vi "Power_ctrl_to_ioEXPSET.vi"(8 "error in (no error)":errorcluster, 10 "IO exp. setting in":u16, 11 "Sensor power control":T1) -> (0 "error out":errorcluster, 2 "Sensor power out":T1, 3 "IO expaneder setting out":u16 format="%x")   [LabVIEW 2013]
doc: "Conversion VI between sent data to control power to sensors and sensor intefaces. \nSet which sensors should be powered in cluster, get coverted bool array using this vi, send to unit.\nGet status from unit, convert it using this VI to cluster where you see which sensors are powered.\n\nBool array is useless, updated to uint16 input/output"
uses:
  Sensor_power_ctrl.ctl
panel:
  out "Boolean array":bool[](array[boolean])
  out "size(s) 2":i32
  out "size(s)":i32
  in  "lookup port":u16[](array[numeric])=[3, 2, 6, 7, 14, 15, 4, 5, 1, 0] format="%0d"
  out "Bool Array out":bool[](array[boolean])
  # "power control to bool array"
  # "index is power control in order\nvalue is specific IOexp output\nordered 0 is 0.0, 7 is 0.7, 8 is 1.0 15 is 1.7"
  # "8"
  # "old values"
  # "bool array to power control"
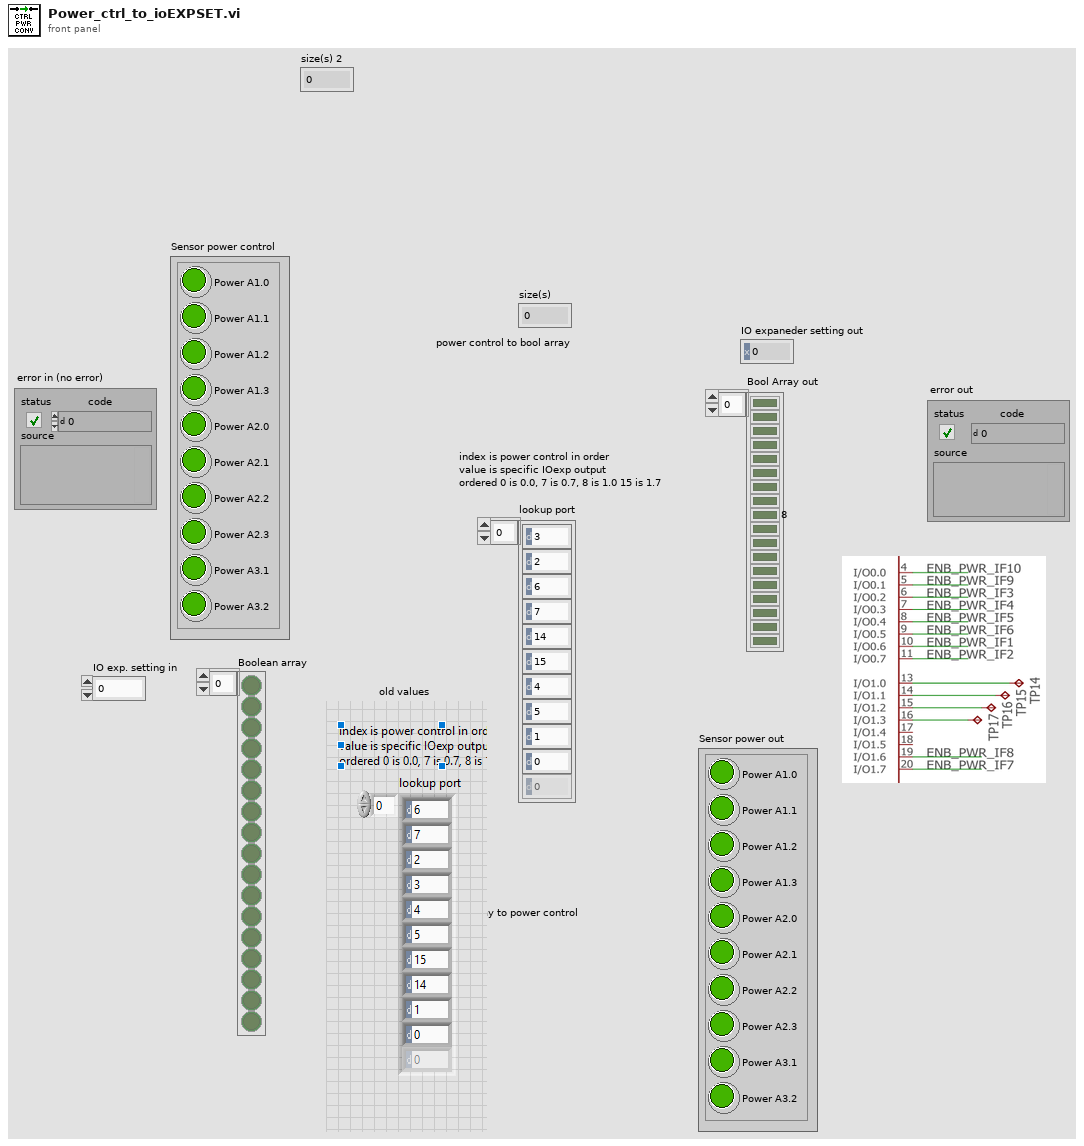
[diagram p1: front panel]
types:
  T1 = typedef "Sensor_power_ctrl.ctl" = cluster{"Power A1.0":bool, "Power A1.1":bool, "Power A1.2":bool, "Power A1.3":bool, "Power A2.0":bool, "Power A2.1":bool, "Power A2.2":bool, "Power A2.3":bool, "Power A3.1":bool, "Power A3.2":bool}
  T2 = cluster{"[0]":bool, "[1]":bool, "[2]":bool, "[3]":bool, "[4]":bool, "[5]":bool, "[6]":bool, "[7]":bool, "[8]":bool, "[9]":bool}
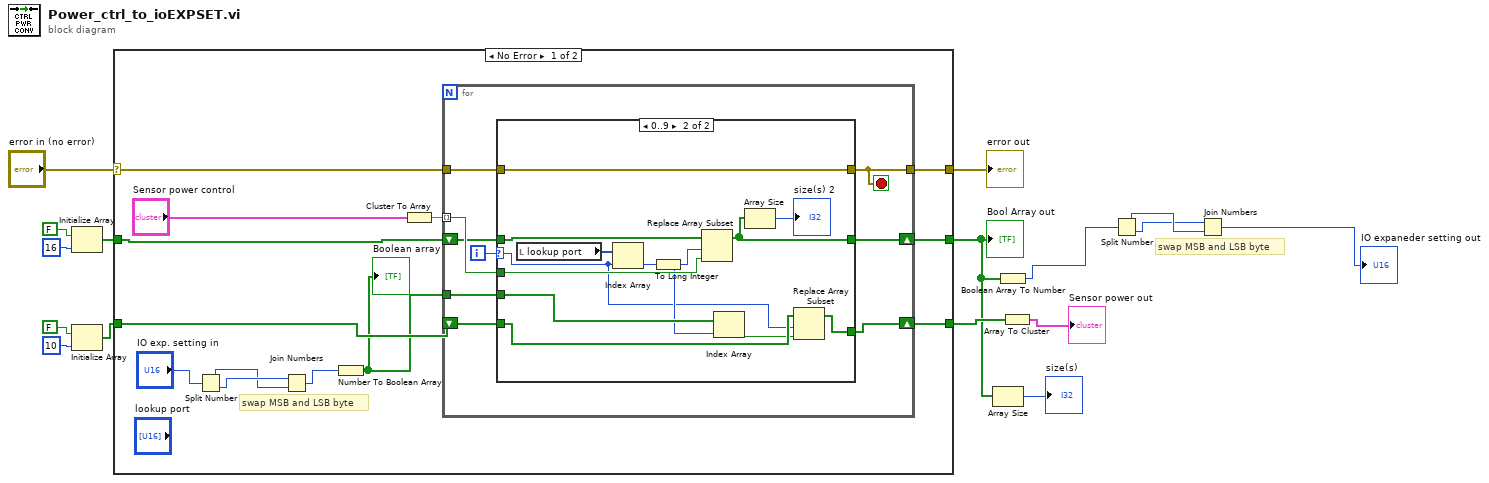
[diagram p0: block diagram]
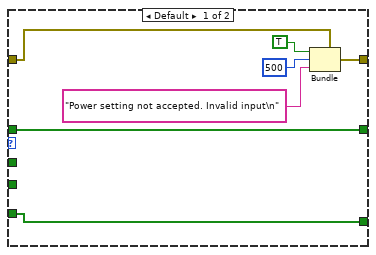
[diagram p2: hidden frame]
diagram:
  # "swap MSB and LSB byte"
  n1 = Initialize Array(FALSE, 16 ("dimension size")) -> (w12:bool[])
  n2 = Initialize Array(FALSE, 10 ("dimension size")) -> (w8:bool[])
  n3 = case shown="No Error" "error in (no error)" {
    selector: "error in (no error)" -> [w29 w60]
    tunnel: [w28 w60] -> w15
    tunnel: w12 -> [w27 _]
    tunnel: [w26 _] -> w5
    tunnel: [w23 w59] -> w7
    tunnel: w8 -> [w22 w59]
    frame No Error {
      # "swap MSB and LSB byte"
      n4 = Split Number(x="IO exp. setting in") -> (hi(x)=w17:u8, lo(x)=w18:u8)
      n5 = Join Numbers(hi=w18, lo=w17) -> ((hi.lo)=w19:u16)
      n6 = Number To Boolean Array(number=w19) -> (Boolean array=w21:bool[])
      "Boolean array" <- w21
      n7 = Cluster To Array(cluster="Sensor power control") -> (array=w25:bool[])
      n8 = for {
        tunnel: w25 -> [w38] mode=indexing
        tunnel: w29 -> [w37]
        tunnel: [w36] -> w28
        shift-right: [w34] -> w26
        shift-left: w27 -> [w35]
        tunnel: w21 -> [w32]
        shift-right: [w31] -> w23
        shift-left: w22 -> [w30]
        i -> [w33]
        stop <- w36 stop-if-true
        n9 = case shown="0..9" w33 {
          selector: w33 -> [_ w46]
          tunnel: w38 -> [_ w53]
          tunnel: [w45 w58] -> w36
          tunnel: w37 -> [w44 w58]
          tunnel: w35 -> [w40 w54]
          tunnel: [w40 w52] -> w34
          tunnel: w32 -> [_ w51]
          tunnel: w30 -> [w39 w48]
          tunnel: [w39 w49] -> w31
          frame Default {
            n10 = Bundle(cluster=w44, "status"=TRUE, "code"=500, "source"="Power setting not accepted. Invalid input\n") -> (w45:errorcluster)
          }
          frame 0..9 {
            n11 = local read "lookup port"() -> (w57:u16[])
            n12 = Index Array(array=w57, index=w46) -> (element=w56:u16)
            n13 = To Long Integer(number=w56) -> (32bit integer=w50:i32)
            n14 = Replace Array Subset(array=w54, new element=w53, index=w50) -> (w52:bool[])
            n15 = Index Array(array=w51, index=w50) -> (element=w47:bool)
            n16 = Array Size(array=w52) -> (size(s)=→"size(s) 2":i32)
            n17 = Replace Array Subset(array=w48, new element=w47, index=w46) -> (w49:bool[])
          }
        }
      }
    }
    frame Error {
    }
  }
  "error out" <- w15
  "Bool Array out" <- w5
  n18 = Array Size(array=w5) -> (size(s)=→"size(s)":i32)
  n19 = Boolean Array To Number(Boolean array=w5) -> (number=w2:u16)
  n20 = Array To Cluster(array=w7) -> (cluster=→"Sensor power out":T2)
  n21 = Split Number(x=w2) -> (hi(x)=w4:u8, lo(x)=w3:u8)
  n22 = Join Numbers(hi=w3, lo=w4) -> ((hi.lo)=→"IO expaneder setting out":u16)
